vi "redovi_argumenti.vi"() -> ()   [LabVIEW 2023]
uses:
  Downloads/Timer/Timer 2013/Control Timer.ctl
panel:
  out "Test":bool
  out "error out":errorcluster
  out "Stanje":string
  in  "stop":bool
  in  "Run Test 2":bool
  in  "Run Test 1":bool
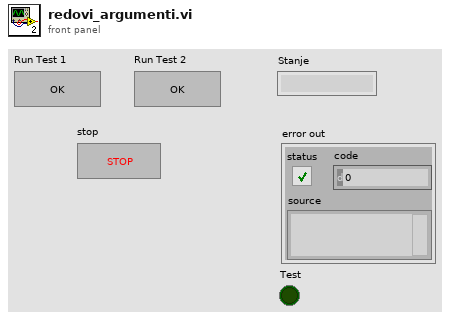
[diagram p1: front panel]
types:
  T1 = typedef "Control Timer.ctl" = enum16{"Timecheck", "Reset"}
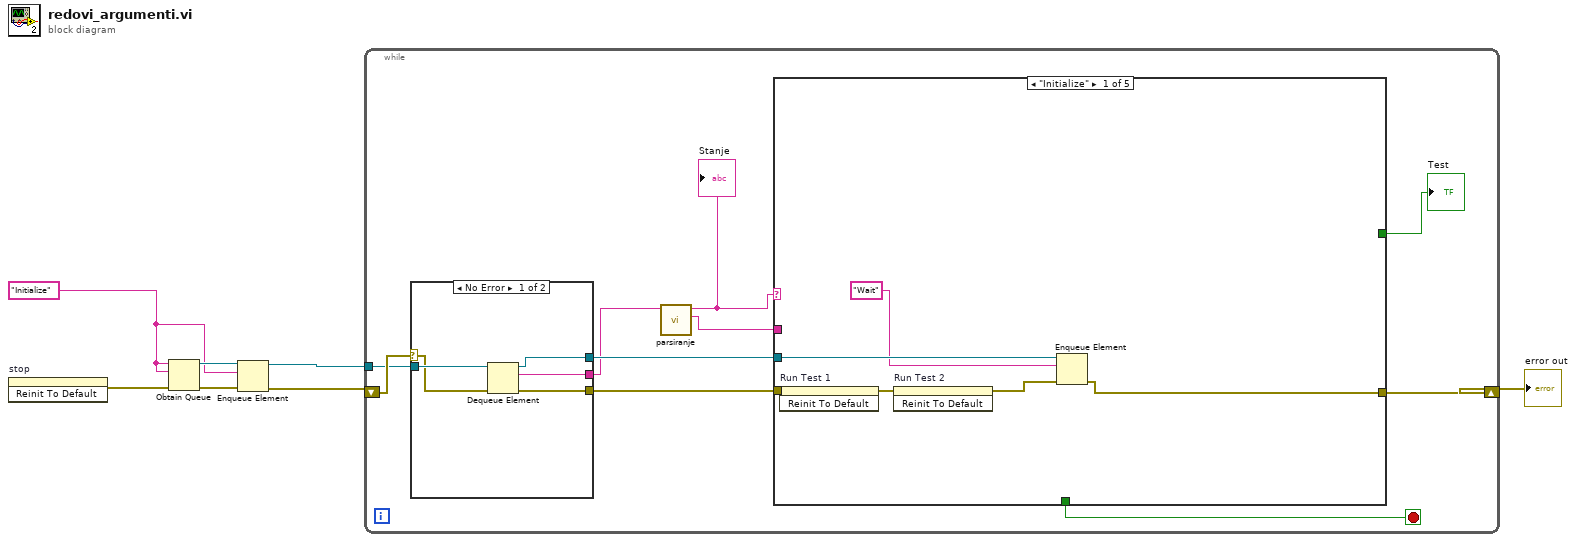
[diagram p0: block diagram]
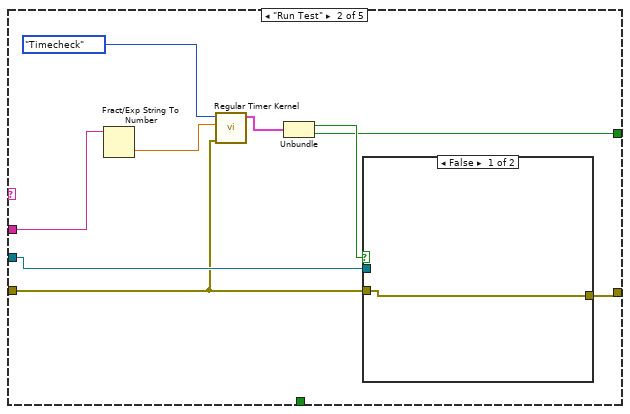
[diagram p2: hidden frame]
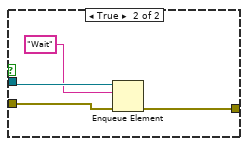
[diagram p3: hidden frame]
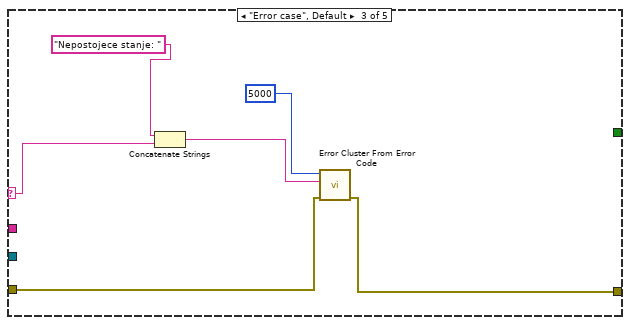
[diagram p4: hidden frame]
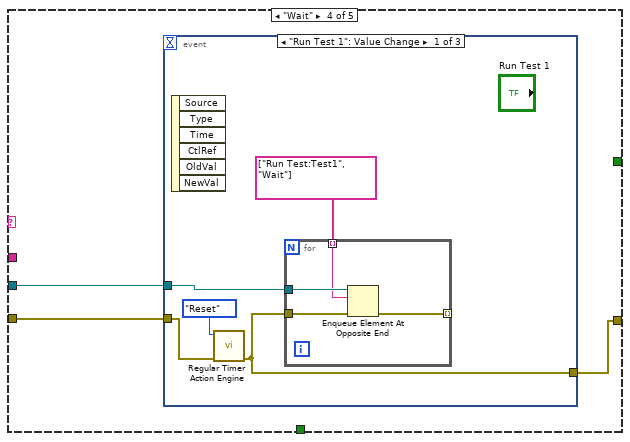
[diagram p5: hidden frame]
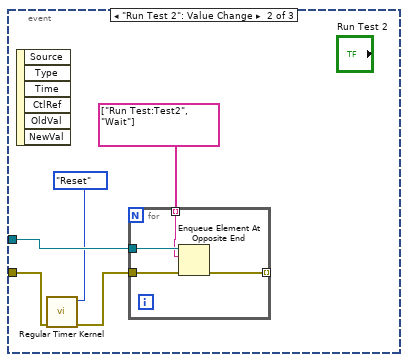
[diagram p6: hidden frame]
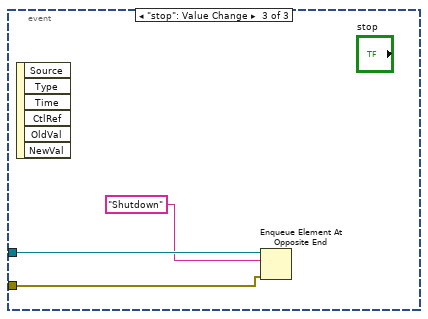
[diagram p7: hidden frame]
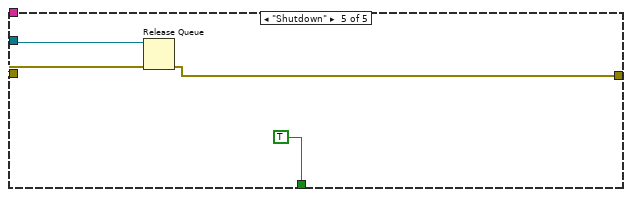
[diagram p8: hidden frame]
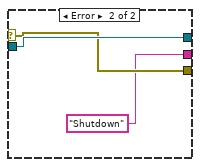
[diagram p9: hidden frame]
diagram:
  w2 = "Initialize"
  n1 = invoke on="stop" class="Bool" method="Reinit To Default"() -> (error out=w5:errorcluster)  [unwired: 3 in, 2 out]
  n2 = Obtain Queue(name (unnamed)=w2, element data type=w2, error in (no error)=w5) -> (queue out=w6:refnum<queue>, error out=w7:errorcluster)  [unwired: 2 in, 1 out]
  n3 = Enqueue Element(queue=w6, element=w2, error in (no error)=w7) -> (queue out=w3:refnum<queue>, error out=w4:errorcluster)  [unwired: 1 in, 1 out]
  n4 = while {
    shift-right: [w9] -> w1
    shift-left: w4 -> [w17]
    tunnel: w3 -> [w16]
    stop <- w13 stop-if-true
    n5 = case shown="No Error" w17 {
      selector: w17 -> [w75 w78]
      tunnel: w16 -> [w76 w79]
      tunnel: [w74 w78] -> w15
      tunnel: [w73 w79] -> w14
      tunnel: [w72 "Shutdown"] -> w12
      frame No Error {
        n6 = Dequeue Element(queue=w76, error in (no error)=w75) -> (queue out=w73:refnum<queue>, element=w72:string, error out=w74:errorcluster)  [unwired: 1 in, 1 out]
      }
      frame Error {
      }
    }
    n7 = call "parsiranje.vi"("Ulaz"=w12) -> ("Argument"=w10:string, "Stanje"=w11:string)  [unwired: 9 in]
    "Stanje" <- w11
    n8 = case shown="\"Initialize\"" w11 {
      selector: w11 -> [_ _ w41 _ _]
      tunnel: w15 -> [w23 w25 w39 w45 w69]
      tunnel: w14 -> [w20 w26 _ w46 w70]
      tunnel: [_ _ _ _ TRUE] -> w13
      tunnel: w10 -> [_ w31 _ _ _]
      tunnel: [w18 w24 w38 w44 w68] -> w9
      tunnel: [_ w27 _ _ _] -> w8
      frame "Initialize" {
        n9 = invoke on="Run Test 1" class="Bool" method="Reinit To Default"(error in=w23) -> (error out=w22:errorcluster)  [unwired: 2 in, 2 out]
        n10 = invoke on="Run Test 2" class="Bool" method="Reinit To Default"(error in=w22) -> (error out=w21:errorcluster)  [unwired: 2 in, 2 out]
        n11 = Enqueue Element(queue=w20, element="Wait", error in (no error)=w21) -> (error out=w18:errorcluster)  [unwired: 1 in, 2 out]
      }
      frame "Run Test" {
        n12 = Fract/Exp String To Number(string=w31) -> (number=w30:dbl)  [unwired: 3 in, 1 out]
        n13 = call "Regular Timer Kernel.vi"("error in"=w25, "Time Target"=w30, "Enum"=Control_Timer."Timecheck") -> ("Status"=w29:cluster{"Running":bool, "Done":bool})  [unwired: 6 in, 2 out]
        n14 = Unbundle(w29) -> ("Running"=w28:bool, "Done"=w27:bool)
        n15 = case shown="False" w28 {
          tunnel: w26 -> [_ w37]
          tunnel: w25 -> [w33 w35]
          tunnel: [w33 w34] -> w24
          frame False {
          }
          frame True {
            n16 = Enqueue Element(queue=w37, element="Wait", error in (no error)=w35) -> (error out=w34:errorcluster)  [unwired: 1 in, 2 out]
          }
        }
      }
      frame "Error case", Default {
        n17 = Concatenate Strings("Nepostojece stanje: ", w41) -> (w40:string)
        n18 = call <vilib>:"Error Cluster From Error Code.vi"("error in (no error)"=w39, "error message (\"\")"=w40, "error code (0)"=5000) -> ("error out"=w38:errorcluster)  [unwired: 6 in]
      }
      frame "Wait" {
        n19 = event shown="[0] \"Run Test 1\": Value Change" {
          selector: _ -> [_ _ _]
          dyn-events: _ -> [_ _ _]
          timeout: _ -> [_ _ _]
          tunnel: w46 -> [w51 w60 w67]
          tunnel: w45 -> [w48 w57 w66]
          tunnel: [w47 _ _] -> w44
          event "Run Test 1": Value Change {
            n20 = event-data() -> ()  [unwired: 1 in, 6 out]
            n21 = call "Regular Timer Action Engine.vi"("Enum"=Control_Timer."Reset", "error in"=w48) -> ("error out"=w47:errorcluster)  [unwired: 7 in, 1 out]
            n22 = for {
              tunnel: w51 -> [w55]
              tunnel: string[] ["Run Test:Test1", "Wait"] -> [w54] mode=indexing
              tunnel: w47 -> [w53]
              tunnel: [w52] -> _ mode=indexing
              n23 = Enqueue Element At Opposite End(queue=w55, element=w54, error in (no error)=w53) -> (error out=w52:errorcluster)  [unwired: 1 in, 2 out]
            }
          }
          event "Run Test 2": Value Change {
            n24 = event-data() -> ()  [unwired: 1 in, 6 out]
            n25 = call "Regular Timer Kernel.vi"("error in"=w57, "Enum"=Control_Timer."Reset") -> ("error out"=w56:errorcluster)  [unwired: 7 in, 2 out]
            n26 = for {
              tunnel: w60 -> [w64]
              tunnel: [w63] -> _ mode=indexing
              tunnel: string[] ["Run Test:Test2", "Wait"] -> [w62] mode=indexing
              tunnel: w56 -> [w61]
              n27 = Enqueue Element At Opposite End(queue=w64, element=w62, error in (no error)=w61) -> (error out=w63:errorcluster)  [unwired: 1 in, 2 out]
            }
          }
          event "stop": Value Change {
            n28 = event-data() -> ()  [unwired: 1 in, 6 out]
            n29 = Enqueue Element At Opposite End(queue=w67, element="Shutdown", error in (no error)=w66) -> ()  [unwired: 1 in, 3 out]
          }
        }
      }
      frame "Shutdown" {
        n30 = Release Queue(queue=w70, error in (no error)=w69) -> (error out=w68:errorcluster)  [unwired: 1 in, 2 out]
      }
    }
    "Test" <- w8
  }
  "error out" <- w1
